vi "Get Template Dut Results.vi"(8 "error in (no error)":errorcluster, 11 "Template Dut in":refnum<class "Template Dut.lvclass">) -> (0 "error out":errorcluster, 2 "Template Dut Results":T1, 3 "Template Dut out":refnum<class "Template Dut.lvclass">)   [LabVIEW 2015, in "niDTS Template.lvlib" / "Template Dut.lvclass"]
uses:
  Template Dut.lvclass
  Includes/Template Dut INC Results.ctl
  Template Dut.lvclass/Template Dut.ctl
  niDTS Template.lvlib
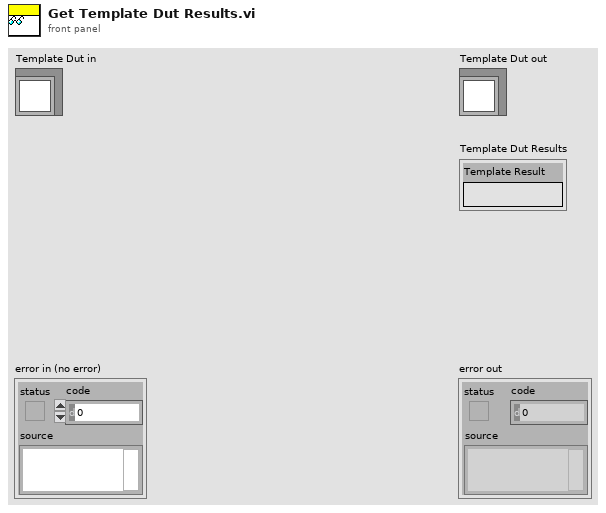
[diagram p1: front panel]
types:
  T1 = typedef "niDTS Template.lvlib/Template Dut INC Results.ctl" = cluster{"Template Result":string}
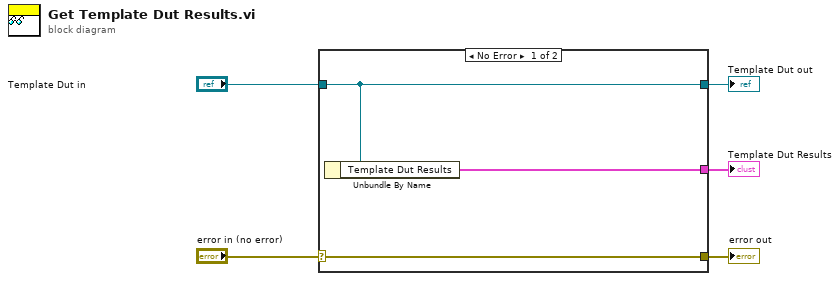
[diagram p0: block diagram]
diagram:
  n1 = case shown="No Error" "error in (no error)" {
    selector: "error in (no error)" -> [w8 w9]
    tunnel: [w8 w9] -> w4
    tunnel: [w7 w10] -> w2
    tunnel: "Template Dut in" -> [w7 w10]
    tunnel: [w6 _] -> w1
    frame No Error {
      n2 = Unbundle By Name(w7) -> ("Template Dut Results"=w6:T1)
    }
    frame Error {
    }
  }
  "error out" <- w4
  "Template Dut out" <- w2
  "Template Dut Results" <- w1
